vi "Calc CRC-16.vi"(3 "Frame in":u8[](array[numeric]) format="%.0x") -> (1 "CRC-16":u8[](array[numeric]) format="%.0x")   [LabVIEW 2012, in "MB Master.lvlib" / "MB_ADU_RTU.lvclass"]
doc: "Calculates the 16-bit CRC of a Modbus RTU ADU (<Address><Function Code><[Data]>)"
uses:
  MB_ADU_RTU.lvclass
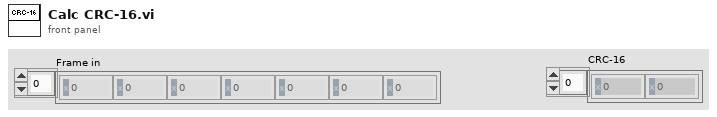
[diagram p1: front panel]
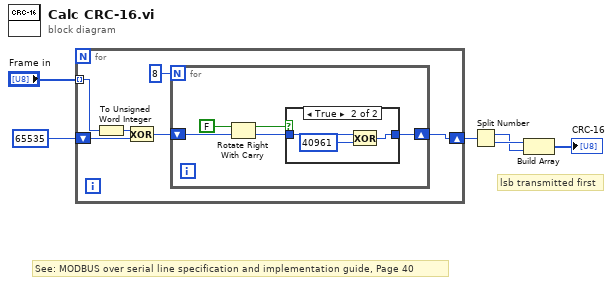
[diagram p0: block diagram]
diagram:
  # "lsb transmitted first"
  # "See: MODBUS over serial line specification and implementation guide, Page 40"
  n1 = for {
    tunnel: "Frame in" -> [w11] mode=indexing
    shift-right: [w7] -> w4
    shift-left: u16 65535 -> [w12]
    n2 = To Unsigned Word Integer(number=w11) -> (unsigned 16bit integer=w10:u16)
    n3 = Exclusive Or(1:w12, 2:w10) -> (0:w8:u16)
    n4 = for {
      N: 8 -> [_]
      shift-right: [w13] -> w7
      shift-left: w8 -> [w16]
      n5 = Rotate Right With Carry(2:w16, 3:FALSE ("carry")) -> (0:w14:u16, 1:w15:bool)
      n6 = case shown="True" w15 {
        tunnel: [w18 w19] -> w13
        tunnel: w14 -> [w18 w20]
        frame False {
        }
        frame True {
          n7 = Exclusive Or(1:u16 40961, 2:w20) -> (0:w19:u16)
        }
      }
    }
  }
  n8 = Split Number(x=w4) -> (hi(x)=w2:u8, lo(x)=w3:u8)
  n9 = Build Array(w3, w2) -> (→"CRC-16":u8[])
